vi "Cal BC (VIRef).vi"(8 "error in (no error)":errorcluster, 10 "BC in":variant, 11 "Domain_Steady_2D_Rect in":refnum<class "NI_Domain_Steady_2D_Rect.lvclass">) -> (0 "error out":errorcluster, 2 "BC out":variant, 3 "Domain_Steady_2D_Rect out":refnum<class "NI_Domain_Steady_2D_Rect.lvclass">)   [LabVIEW 2017, in "NI_PDE.lvlib" / "NI_Domain_Steady_2D_Rect.lvclass"]
uses:
  <vilib>/gmath/pde.llb/DomainClass/Domain_Steady_2D_Rect/NI_Domain_Steady_2D_Rect.lvclass
  <vilib>/gmath/pde.llb/Common/PDE_BC Position 2D.ctl
  <vilib>/gmath/pde.llb/BCClass/BC_Steady_2D_VIRef/BC Data.ctl
  <vilib>/gmath/pde.llb/Common/PDE_BC Type.ctl
  <vilib>/gmath/pde.llb/BCClass/BC_Steady_2D_Numeric/BC Data.ctl
  <vilib>/gmath/pde.llb/DomainClass/Domain_Steady_2D_Rect/NI_Domain_Steady_2D_Rect.lvclass/NI_Domain_Steady_2D_Rect.ctl
  <vilib>/Analysis/1siggen.llb/Ramp Pattern by Samples.vi
  <vilib>/gmath/NI_PDE.lvlib
  <vilib>/gmath/pde.llb/BCClass/BC_Steady_2D_VIRef/NI_BC_Steady_2D_VIRef.lvclass
  <vilib>/gmath/pde.llb/BCClass/BC_Steady_2D_Numeric/NI_BC_Steady_2D_Numeric.lvclass
  <vilib>/Analysis/NI_AALBase.lvlib
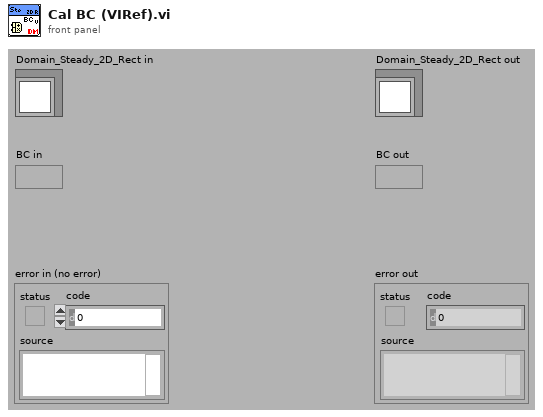
[diagram p1: front panel]
types:
  T1 = typedef "NI_PDE.lvlib/NI_BC_Steady_2D_Numeric.lvclass/BC Data.ctl" = cluster{"type":T2, "position":T3, "G":dbl[]}
  T2 = typedef "NI_PDE.lvlib/PDE_BC Type.ctl" = i32
  T3 = typedef "NI_PDE.lvlib/PDE_BC Position 2D.ctl" = i32
  T4 = typedef "NI_PDE.lvlib/NI_BC_Steady_2D_VIRef.lvclass/BC Data.ctl" = cluster{"type":T2, "position":T3, "G":refnum<vi>, "data":variant}
  T5 = cluster{"start x":dbl, "end x":dbl, "# of x-points":i32}
  T6 = cluster{"start y":dbl, "end y":dbl, "# of y-points":i32}
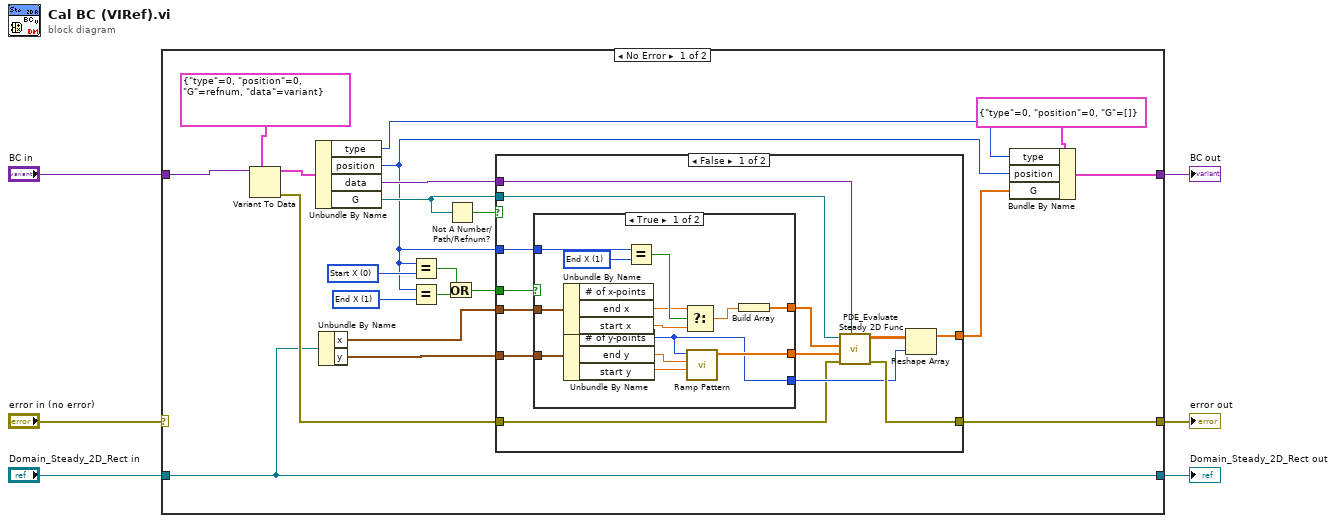
[diagram p0: block diagram]
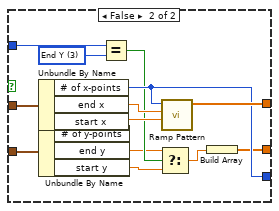
[diagram p2: hidden frame]
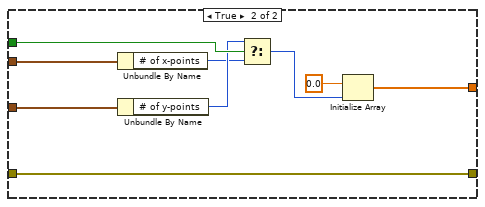
[diagram p3: hidden frame]
diagram:
  n1 = case shown="No Error" "error in (no error)" {
    selector: "error in (no error)" -> [_ w78]
    tunnel: "Domain_Steady_2D_Rect in" -> [w7 w77]
    tunnel: [w7 w77] -> w6
    tunnel: [w16 w78] -> w5
    tunnel: [w14 w76] -> w2
    tunnel: "BC in" -> [w19 w76]
    frame No Error {
      w26 = T3 1 items=["Start X", "End X", "Start Y", "End Y"] ("y")
      w27 = T3 0 items=["Start X", "End X", "Start Y", "End Y"] ("y")
      n2 = Variant To Data(type=T4 {"type"=0, "position"=0, "G"=refnum, "data"=variant} ("BC data"), Variant=w19) -> (data=w17:T4, error out=w8:errorcluster)  [unwired: 1 in]
      n3 = Unbundle By Name(w17) -> ("type"=w12:T2, "position"=w11:T3, "data"=w20:variant, "G"=w21:refnum<vi>)
      n4 = Unbundle By Name(w7) -> ("x"=w10:T5, "y"=w9:T6)
      n5 = Equal?(x=w11, y=w27) -> (x = y?=w25:bool)
      n6 = Equal?(x=w11, y=w26) -> (x = y?=w24:bool)
      n7 = Or(x=w25, y=w24) -> (x .or. y?=w23:bool)
      n8 = Not A Number/Path/Refnum?(number/path/refnum=w21) -> (NaN/Path/Refnum?=w22:bool)
      n9 = case shown="False" w22 {
        tunnel: [w33 w75] -> w13
        tunnel: w10 -> [w39 w74]
        tunnel: w9 -> [w30 w73]
        tunnel: w23 -> [w40 w71]
        tunnel: w8 -> [w28 w67]
        tunnel: [w38 w67] -> w16
        tunnel: w21 -> [w36 _]
        tunnel: w20 -> [w35 _]
        tunnel: w11 -> [w31 _]
        frame False {
          n10 = case shown="True" w40 {
            tunnel: w39 -> [w47 w59]
            tunnel: [w43 w62] -> w37
            tunnel: [w41 w61] -> w32
            tunnel: w31 -> [w51 w66]
            tunnel: w30 -> [w48 w58]
            tunnel: [w42 w54] -> w29
            frame True {
              w50 = T3 1 items=["Start X", "End X", "Start Y", "End Y"] ("y")
              n11 = Unbundle By Name(w47) -> ("end x"=w46:dbl, "start x"=w45:dbl)  [unwired: 1 out]
              n12 = Unbundle By Name(w48) -> ("# of y-points"=w41:i32, "end y"=w52:dbl, "start y"=w53:dbl)
              n13 = Equal?(x=w51, y=w50) -> (x = y?=w49:bool)
              n14 = Select(t=w46, s=w49, f=w45) -> (s? t:f=w44:dbl)
              n15 = call-poly <vilib>:"Ramp Pattern.vi"("start"=w53, "end"=w52, "samples"=w41) -> ("Ramp Pattern"=w42:dbl[])  [unwired: 7 in, 1 out]
              n16 = Build Array(w44) -> (w43:dbl[])
            }
            frame False {
              w65 = T3 3 items=["Start X", "End X", "Start Y", "End Y"] ("y")
              n17 = Unbundle By Name(w59) -> ("# of x-points"=w61:i32, "end x"=w63:dbl, "start x"=w64:dbl)
              n18 = Unbundle By Name(w58) -> ("end y"=w57:dbl, "start y"=w56:dbl)  [unwired: 1 out]
              n19 = Equal?(x=w66, y=w65) -> (x = y?=w60:bool)
              n20 = Select(t=w57, s=w60, f=w56) -> (s? t:f=w55:dbl)
              n21 = call-poly <vilib>:"Ramp Pattern.vi"("start"=w64, "end"=w63, "samples"=w61) -> ("Ramp Pattern"=w62:dbl[])  [unwired: 7 in, 1 out]
              n22 = Build Array(w55) -> (w54:dbl[])
            }
          }
          n23 = call <vilib>:"PDE_Evaluate Steady 2D Func.vi"("data"=w35, "error in (no error)"=w28, "Y"=w29, "X"=w37, "VIRef"=w36) -> ("error out"=w38:errorcluster, "F(x, y)"=w34:dbl[][])  [unwired: 5 out]
          n24 = Reshape Array(w34, w32) -> (w33:dbl[])
        }
        frame True {
          n25 = Unbundle By Name(w74) -> ("# of x-points"=w68:i32)
          n26 = Unbundle By Name(w73) -> ("# of y-points"=w70:i32)
          n27 = Select(t=w70, s=w71, f=w68) -> (s? t:f=w69:i32)
          n28 = Initialize Array(0.0 ("element"), w69) -> (w75:dbl[])
        }
      }
      n29 = Bundle By Name(cluster=T1 {"type"=0, "position"=0, "G"=[]} ("BC data"), "type"=w12, "position"=w11, "G"=w13) -> (w14:T1)
    }
    frame Error {
    }
  }
  "Domain_Steady_2D_Rect out" <- w6
  "error out" <- w5
  "BC out" <- w2
